vi "pulse duration to duty cycle.vi"(10 "Pulse duration Laser  (ms)":dbl, 11 "frequency":dbl) -> (3 "% duty cyle":dbl)   [LabVIEW 2015]
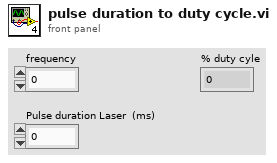
[diagram p1: front panel]
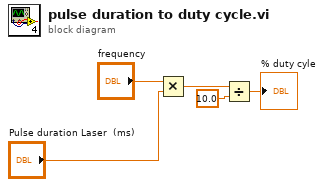
[diagram p0: block diagram]
diagram:
  n1 = Multiply(x="frequency", y="Pulse duration Laser  (ms)") -> (x*y=w3:dbl)
  n2 = Divide(x=w3, y=10.0) -> (x/y=→"% duty cyle":dbl)
